vi "Destroy.vi"(0 "reference in":refnum<class "DataGridView.lvclass">, 11 "error in (no error)":errorcluster) -> (4 "reference out":refnum<class "DataGridView.lvclass">, 15 "error out":errorcluster)   [LabVIEW 2018, in "DataGridView.lvclass"]
uses:
  DataGridView.lvclass
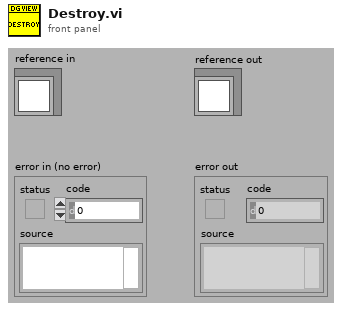
[diagram p1: front panel]
types:
  T1 = typedef "DataGridView.lvclass/ObjectAttributes.ctl" = cluster{"DataGridView":refnum<k24>, "SelectionChangedEvent":refnum<user-event>, "SelectionChanged callback ref":refnum<k27>, "LastSelectedRowIndex":i32, "CellClickEvent":refnum<user-event>, "CellClick callback refnum":refnum<k27>}
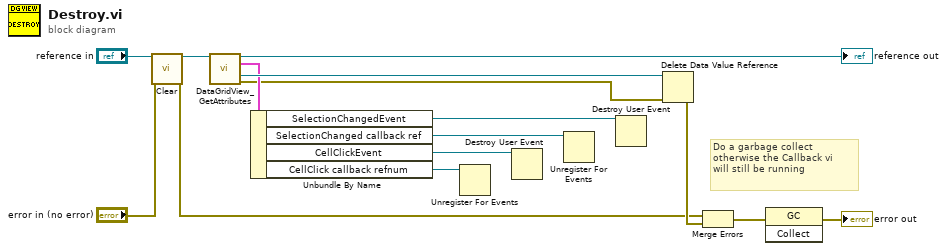
[diagram p0: block diagram]
diagram:
  # "Do a garbage collect otherwise the Callback vi \nwill still be running"
  n1 = call-dynamic "Clear.vi"("reference in"="reference in", "error in (no error)"="error in (no error)") -> ("reference out"=w9:refnum<class "DataGridView.lvclass">, "error out"=w7:errorcluster)  [unwired: 12 in]
  n2 = call "DataGridView_GetAttributes.vi"("reference in"=w9) -> ("reference out"=→"reference out":refnum<class "DataGridView.lvclass">, "Data"=w12:T1, "DataRef"=w13:refnum<data-value>, "error out"=w1:errorcluster)  [unwired: 11 in]
  n3 = Unbundle By Name(w12) -> ("SelectionChangedEvent"=w10:refnum<user-event>, "SelectionChanged callback ref"=w4:refnum<k27>, "CellClickEvent"=w2:refnum<user-event>, "CellClick callback refnum"=w3:refnum<k27>)
  n4 = Unregister For Events(event registration refnum=w3) -> ()  [unwired: 1 in, 1 out]
  n5 = Destroy User Event(user event=w2) -> ()  [unwired: 1 in, 1 out]
  n6 = Unregister For Events(event registration refnum=w4) -> ()  [unwired: 1 in, 1 out]
  n7 = Destroy User Event(user event=w10) -> ()  [unwired: 1 in, 1 out]
  n8 = Delete Data Value Reference(data value reference=w13, error in=w1) -> (error out=w11:errorcluster)  [unwired: 1 out]
  n9 = Merge Errors(w7, w11) -> (w6:errorcluster)
  n10 = invoke class="GC" method="Collect"(error in=w6) -> (error out=→"error out":errorcluster)  [unwired: 2 in, 2 out]
